vi "WSVCAP SHL Host LL RFFE Write.vi"(0 "RTFFE Data":u8[][](array[numeric]) format="%.0x", 1 "Wait Ticks":u32, 2 "Slave Address":u8, 5 "Socket Mask":u64=1 format="%02x", 7 "Cycle CMD Lengths Out (bits)":u8[](array[numeric]), 9 "Cycle CMD Delay Out (ticks)":u32[](array[numeric]), 11 "error in":errorcluster, 14 "FPGA":T1) -> (8 "Status":u8[](array[numeric]), 15 "error out":errorcluster)   [LabVIEW 2017]
uses:
  Type Defs/WSVCAP SHL FPGA Enum.ctl
  Type Defs/WSVCAP SHL Top Level Write Read State Enum.ctl
  Type Defs/WSVCAP SHL State.ctl
  Type Defs/WSVCAP SHL Top Level Control Enum.ctl
  Type Defs/WSVCAP SHL Transaction Enum.ctl
panel:
  out "Write Data":u64[](array[numeric]) format="%032b"
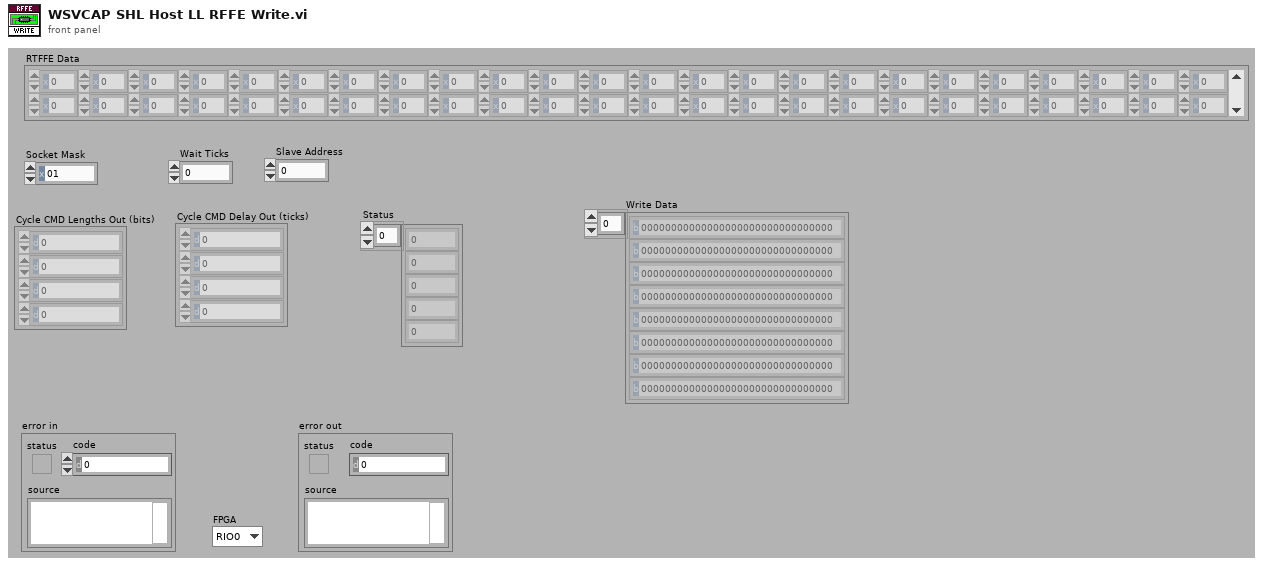
[diagram p1: front panel]
types:
  T1 = typedef "WSVCAP SHL FPGA Enum.ctl" = enum16{"RIO0", "RIO1"}
  T2 = typedef "WSVCAP SHL Top Level Write Read State Enum.ctl" = enum16{"Start", "Write", "Read", "Get Status", "Wait Until Done"}
  T3 = typedef "WSVCAP SHL State.ctl" = enum8{"Idle", "Transfer Data"}
  T4 = typedef "WSVCAP SHL Transaction Enum.ctl" = enum16{"I2C-Read Data", "I2C-Write Data", "RFFE-Ext Write", "RFFE-Ext Read"}
  T5 = typedef "WSVCAP SHL Top Level Control Enum.ctl" = enum16{"Start", "Cmd", "Transaction", "Wait Ticks", "Socket Mask", "UUT Set", "Slave Address", "Sub Address", "Bytes to Write", "Bytes to Read", "Write Data", "Write Flag", "Read Data", "Read Flag", "Ack Read", "Read Status Flag", "Ack Read Status", "Status", "Cycle Count", "Stop Cycle", "Exit"}
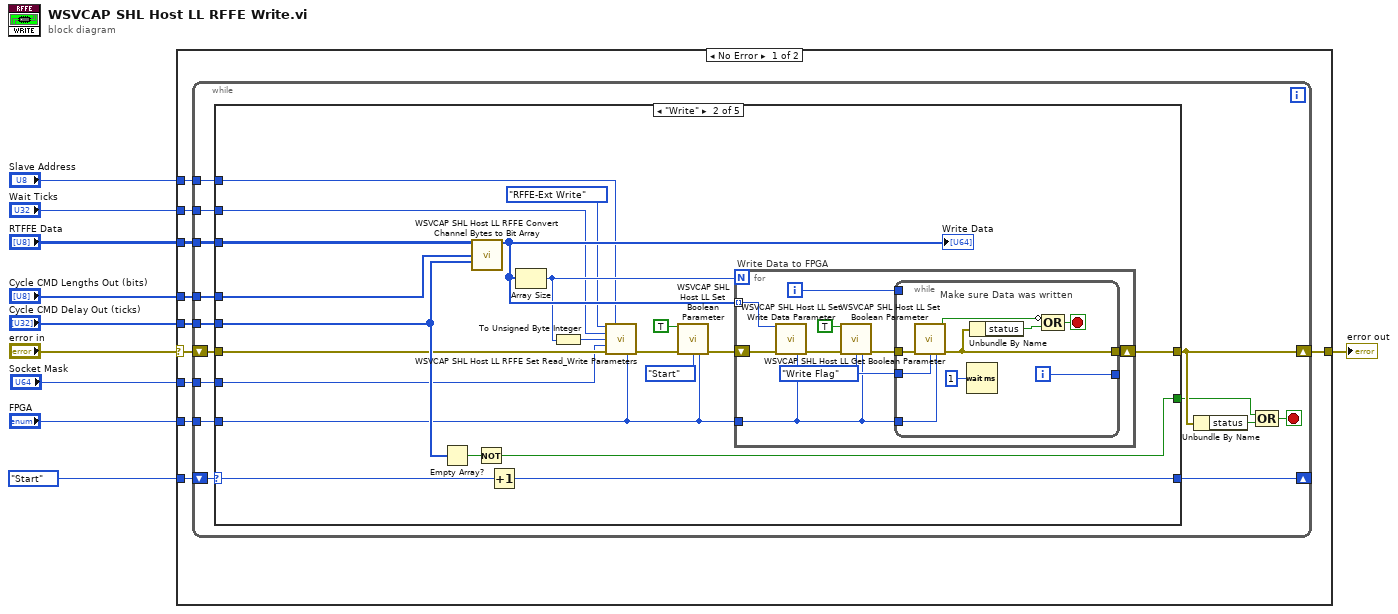
[diagram p0: block diagram]
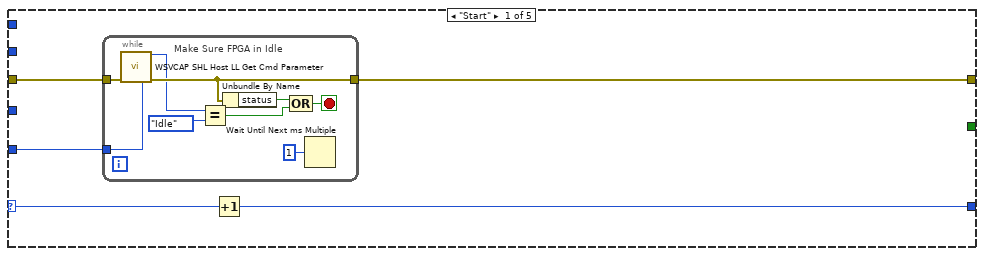
[diagram p2: hidden frame]
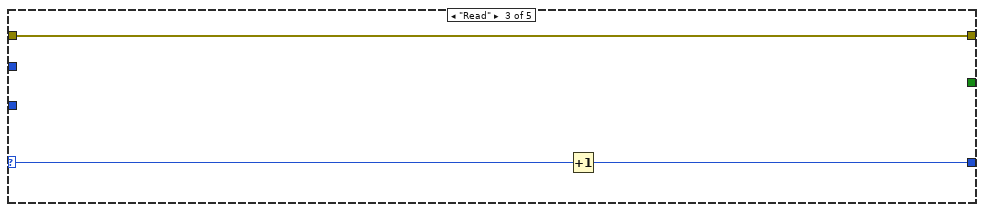
[diagram p3: hidden frame]
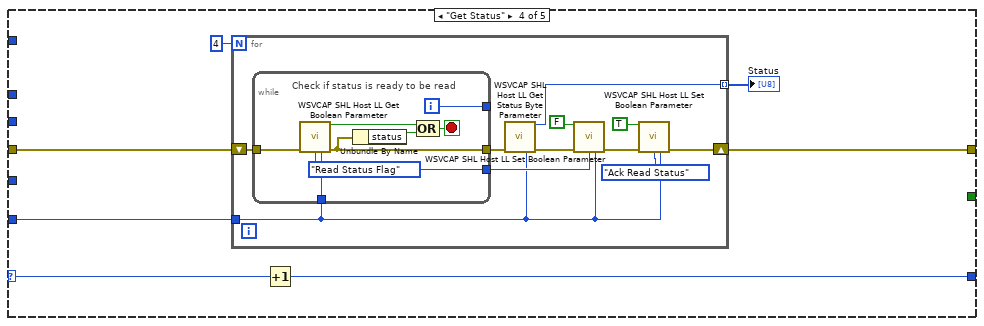
[diagram p4: hidden frame]
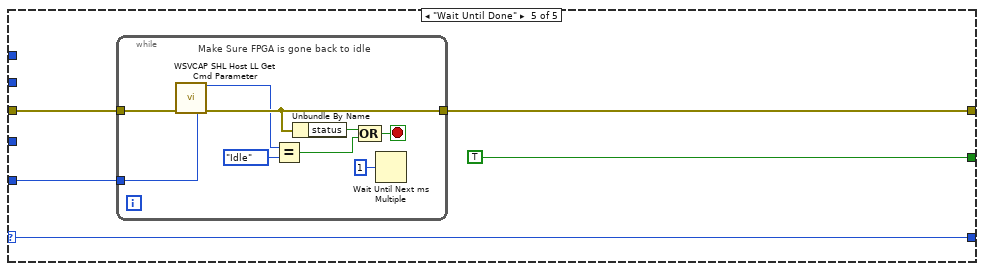
[diagram p5: hidden frame]
diagram:
  n1 = case shown="No Error" "error in" {
    selector: "error in" -> [w16 w131]
    tunnel: [w20 w131] -> w10
    tunnel: WSVCAP_SHL_Top_Level_Write_Read_State_Enum."Start" ("Write Read State") -> [w19 _]
    tunnel: "RTFFE Data" -> [w18 _]
    tunnel: "Socket Mask" -> [w17 _]
    tunnel: "Cycle CMD Lengths Out (bits)" -> [w15 _]
    tunnel: "Cycle CMD Delay Out (ticks)" -> [w14 _]
    tunnel: "Wait Ticks" -> [w13 _]
    tunnel: "Slave Address" -> [w12 _]
    tunnel: "FPGA" -> [w11 _]
    frame No Error {
      n2 = while {
        shift-right: [w33] -> w20
        shift-left: w16 -> [w34]
        shift-right: [w28] -> _
        shift-left: w19 -> [w29]
        tunnel: w18 -> [w27]
        tunnel: w17 -> [w26]
        tunnel: w15 -> [w25]
        tunnel: w14 -> [w24]
        tunnel: w13 -> [w23]
        tunnel: w12 -> [w22]
        tunnel: w11 -> [w21]
        stop <- w30 stop-if-true
        n3 = case shown="\"Write\"" w29 {
          selector: w29 -> [w38 w68 w90 w95 w119]
          tunnel: w34 -> [w39 w57 w88 w97 w121]
          tunnel: [w36 w69 w88 w96 w120] -> w33
          tunnel: [_ w62 _ _ TRUE] -> w32
          tunnel: [w37 w66 w89 w94 w119] -> w28
          tunnel: w27 -> [_ w53 _ _ _]
          tunnel: w26 -> [_ w54 _ _ _]
          tunnel: w25 -> [_ w65 _ _ _]
          tunnel: w24 -> [_ w64 _ _ _]
          tunnel: w23 -> [_ w52 _ _ _]
          tunnel: w22 -> [_ w50 _ _ _]
          tunnel: w21 -> [w35 w49 _ w91 w117]
          frame "Start" {
            n4 = while {
              tunnel: w39 -> [w44]
              tunnel: [w43] -> w36
              tunnel: w35 -> [w40]
              stop <- w48 stop-if-true
              # "Make Sure FPGA in Idle"
              n5 = call "WSVCAP SHL Host LL Get Cmd Parameter.vi"("error in (no error)"=w44, "FPGA"=w40) -> ("I2C_Cmd"=w42:T3, "error out"=w43:errorcluster)  [unwired: 12 in]
              n6 = Equal?(x=w42, y=WSVCAP_SHL_State."Idle" ("Type")) -> (x = y?=w46:bool)
              n7 = Unbundle By Name(w43) -> ("status"=w41:bool)
              n8 = Compound Arithmetic op=OR(w41, w46) -> (w48:bool)
              n9 = Wait Until Next ms Multiple(millisecond multiple=u32 1) -> ()  [unwired: 1 out]
            }
            n10 = Increment(x=w38) -> (x+1=w37:T2)
          }
          frame "Write" {
            # "Write Data to FPGA"
            n11 = Empty Array?(array=w64) -> (empty?=w63:bool)
            n12 = call "WSVCAP SHL Host LL RFFE Convert Channel Bytes to Bit Array.vi"("RFFE Data"=w53, "Cycle CMD Lengths Out (bits)"=w65, "Cycle CMD Delay Out (ticks)"=w64) -> ("Write Data"=w67:u64[])  [unwired: 12 in]
            "Write Data" <- w67
            n13 = Not(x=w63) -> (.not. x?=w62:bool)
            n14 = Increment(x=w68) -> (x+1=w66:T2)
            n15 = Array Size(array=w67) -> (size(s)=w55:i32)
            n16 = To Unsigned Byte Integer(number=w55) -> (unsigned 8bit integer=w58:u8)
            n17 = call "WSVCAP SHL Host LL RFFE Set Read_Write Parameters.vi"("Transaction"=WSVCAP_SHL_Transaction_Enum."RFFE-Ext Write", "Slave Address"=w50, "Wait Ticks"=w52, "Bytes to Write"=w58, "Socket Mask [U64]"=w54, "error in (no error)"=w57, "FPGA"=w49) -> ("error out"=w61:errorcluster)  [unwired: 8 in]
            n18 = call "WSVCAP SHL Host LL Set Boolean Parameter.vi"("Boolean In"=TRUE, "error in (no error)"=w61, "FPGA Top Level Control"=WSVCAP_SHL_Top_Level_Control_Enum."Start", "FPGA"=w49) -> ("error out"=w56:errorcluster)  [unwired: 11 in]
            n19 = for {
              N: w55 -> [_]
              shift-right: [w78] -> w69
              shift-left: w56 -> [w77]
              tunnel: w67 -> [w76] mode=indexing
              tunnel: w49 -> [w70]
              i -> [w71]
              w72 = WSVCAP_SHL_Top_Level_Control_Enum."Write Flag" ("FPGA Top Level Control")
              n20 = call "WSVCAP SHL Host LL Set Write Data Parameter.vi"("Write Byte In"=w76, "error in (no error)"=w77, "FPGA"=w70) -> ("error out"=w75:errorcluster)  [unwired: 12 in]
              n21 = call "WSVCAP SHL Host LL Set Boolean Parameter.vi"("Boolean In"=TRUE, "error in (no error)"=w75, "FPGA Top Level Control"=w72, "FPGA"=w70) -> ("error out"=w73:errorcluster)  [unwired: 11 in]
              n22 = while {
                tunnel: w73 -> [w85]
                tunnel: [w84] -> w78
                tunnel: w72 -> [w82]
                tunnel: w71 -> [_]
                tunnel: [w80] -> _
                tunnel: w70 -> [w79]
                i -> [w80]
                stop <- w87 stop-if-true
                # "Make sure Data was written"
                n23 = call "WSVCAP SHL Host LL Get Boolean Parameter.vi"("error in (no error)"=w85, "FPGA Top Level Control"=w82, "FPGA"=w79) -> ("Boolean Out"=w83:bool, "error out"=w84:errorcluster)  [unwired: 11 in]
                n24 = Wait (ms)(milliseconds to wait=u32 1) -> ()  [unwired: 1 out]
                n25 = Unbundle By Name(w84) -> ("status"=w81:bool)
                n26 = Compound Arithmetic op=OR(invert w83, w81) -> (w87:bool)
              }
            }
          }
          frame "Read" {
            n27 = Increment(x=w90) -> (x+1=w89:T2)
          }
          frame "Get Status" {
            n28 = for {
              N: 4 -> [_]
              shift-right: [w107] -> w96
              shift-left: w97 -> [w108]
              tunnel: [w99] -> w92 mode=indexing
              tunnel: w91 -> [w98]
              n29 = while {
                tunnel: w108 -> [w114]
                tunnel: [w113] -> w106
                tunnel: [w111] -> w104
                tunnel: [w110] -> _
                tunnel: w98 -> [w109]
                i -> [w110]
                stop <- w116 stop-if-true
                w111 = WSVCAP_SHL_Top_Level_Control_Enum."Read Status Flag" ("FPGA Top Level Control")
                # "Check if status is ready to be read"
                n30 = call "WSVCAP SHL Host LL Get Boolean Parameter.vi"("error in (no error)"=w114, "FPGA Top Level Control"=w111, "FPGA"=w109) -> ("Boolean Out"=w115:bool, "error out"=w113:errorcluster)  [unwired: 11 in]
                n31 = Unbundle By Name(w113) -> ("status"=w112:bool)
                n32 = Compound Arithmetic op=OR(w115, w112) -> (w116:bool)
              }
              n33 = call "WSVCAP SHL Host LL Get Status Byte Parameter.vi"("error in (no error)"=w106, "FPGA"=w98) -> ("I2C Status Byte"=w99:u8, "error out"=w105:errorcluster)  [unwired: 12 in]
              n34 = call "WSVCAP SHL Host LL Set Boolean Parameter.vi"("Boolean In"=FALSE ("Read Flag"), "error in (no error)"=w105, "FPGA Top Level Control"=w104, "FPGA"=w98) -> ("error out"=w100:errorcluster)  [unwired: 11 in]
              n35 = call "WSVCAP SHL Host LL Set Boolean Parameter.vi"("Boolean In"=TRUE ("Write Flag"), "error in (no error)"=w100, "FPGA Top Level Control"=WSVCAP_SHL_Top_Level_Control_Enum."Ack Read Status", "FPGA"=w98) -> ("error out"=w107:errorcluster)  [unwired: 11 in]
            }
            "Status" <- w92
            n36 = Increment(x=w95) -> (x+1=w94:T2)
          }
          frame "Wait Until Done" {
            n37 = while {
              tunnel: w121 -> [w125]
              tunnel: [w124] -> w120
              tunnel: w117 -> [w122]
              stop <- w127 stop-if-true
              # "Make Sure FPGA is gone back to idle"
              n38 = call "WSVCAP SHL Host LL Get Cmd Parameter.vi"("error in (no error)"=w125, "FPGA"=w122) -> ("I2C_Cmd"=w123:T3, "error out"=w124:errorcluster)  [unwired: 12 in]
              n39 = Equal?(x=w123, y=WSVCAP_SHL_State."Idle") -> (x = y?=w128:bool)
              n40 = Unbundle By Name(w124) -> ("status"=w129:bool)
              n41 = Compound Arithmetic op=OR(w129, w128) -> (w127:bool)
              n42 = Wait Until Next ms Multiple(millisecond multiple=u32 1) -> ()  [unwired: 1 out]
            }
          }
        }
        n43 = Unbundle By Name(w33) -> ("status"=w31:bool)
        n44 = Compound Arithmetic op=OR(w32, w31) -> (w30:bool)
      }
    }
    frame Error {
    }
  }
  "error out" <- w10
